vi "ENPH 354 Assignment 1 - Q7.vi"() -> ()   [LabVIEW 2021]
panel:
  out "Array":bool[](array[boolean])
  in  "Array 2":bool[](array[boolean])
  in  "Array 1":bool[](array[boolean])
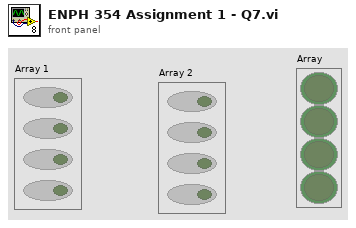
[diagram p1: front panel]
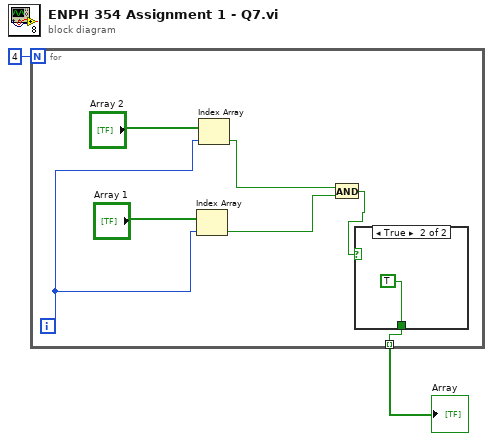
[diagram p0: block diagram]
diagram:
  n1 = for {
    N: 4 -> [_]
    tunnel: [w3] -> w1 mode=indexing
    i -> [w7]
    n2 = Index Array(array="Array 1", index=w7) -> (element=w5:bool)
    n3 = Index Array(array="Array 2", index=w7) -> (element=w4:bool)
    n4 = And(x=w4, y=w5) -> (x .and. y?=w6:bool)
    n5 = case shown="True" w6 {
      tunnel: [_ TRUE] -> w3
      frame False {
      }
      frame True {
      }
    }
  }
  "Array" <- w1
